vi "Increment file number.vi"(8 "error in":errorcluster, 11 "path":path) -> (0 "error out":errorcluster, 3 "path out":path)   [LabVIEW 2013, in "h5logger.lvlib"]
uses:
  h5logger.lvlib
  <vilib>/regexp/Match Regular Expression.xnode
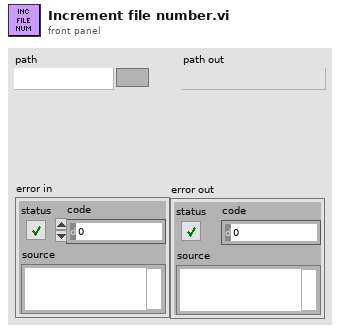
[diagram p1: front panel]
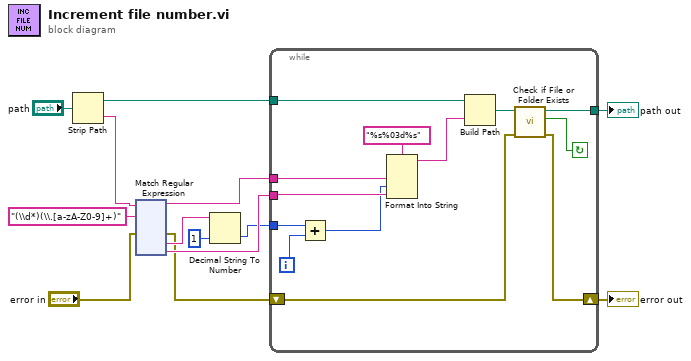
[diagram p0: block diagram]
diagram:
  n1 = Strip Path(path="path") -> (stripped path=w12:path, name=w8:string)
  n2 = xnode "Match Regular Expression"("input string"=w8, "regular expression"="(\\d*)(\\.[a-zA-Z0-9]+)", "error in"="error in") -> ("before match"=w7:string, "error out"=w2:errorcluster, "submatch 1"=w5:string, "submatch 2"=w6:string)  [unwired: 3 in, 3 out]
  n3 = Decimal String To Number(string=w5, default (0L)=1 ("default (0 I32)")) -> (number=w1:i32)  [unwired: 1 in, 1 out]
  n4 = while {
    tunnel: w12 -> [w22]
    tunnel: w7 -> [w24]
    tunnel: w6 -> [w23]
    tunnel: [w18] -> w10
    shift-right: [w17] -> w11
    shift-left: w2 -> [w16]
    tunnel: w1 -> [w15]
    i -> [w26]
    stop <- w19 continue-if-true
    n5 = Add(x=w15, y=w26) -> (x+y=w14:i32)
    n6 = Format Into String(format string="%s%03d%s", w24, w14, w23) -> (resulting string=w21:string)  [unwired: 2 in, 1 out]
    n7 = Build Path(base path=w22, name or relative path=w21) -> (appended path=w20:path)
    n8 = call <vilib>:"Check if File or Folder Exists.vi"("error in (no error)"=w16, "path"=w20) -> ("error out"=w17:errorcluster, "file or folder exists?"=w19:bool, "dup path"=w18:path)  [unwired: 7 in]
  }
  "error out" <- w11
  "path out" <- w10
